vi "HTTP parse headers.vi"(11 "HTTP headers":string="HTTP/1.1 409 Conflict\r\nAccess-Control-Allow-Headers: Origin, X-Requested-With, Content-Type, Accept\r\nAccess-Control-Allow-Methods: GET, POST, PUT, DELETE\r\nAccess-Control-Allow-Origin: *\r\nAccess-Control-Max-Age: 2592000\r\nContent-Type: text/plain\r\nX-Influxdb-Version: InfluxDB v0.8.8 (git: afde71e) (leveldb: 1.15)\r\nDate: Thu, 23 Apr 2015 18:50:38 GMT\r\nContent-Length: 21\r\n\r\n") -> (1 "Status":string, 2 "Status code":string, 3 "HTTP version":string)   [LabVIEW 2013, in "InfluxDB Client.lvclass"]
doc: "Parse HTTP headers to retrieve status information."
uses:
  InfluxDB Client.lvclass
  <vilib>/regexp/Match Regular Expression.xnode
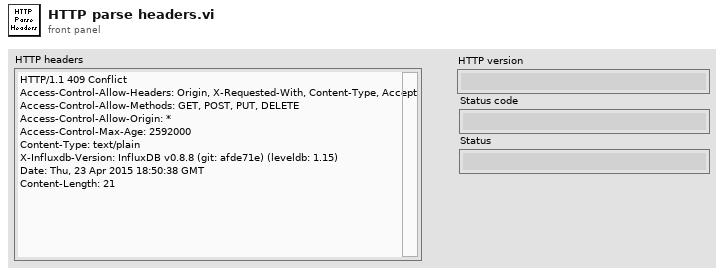
[diagram p1: front panel]
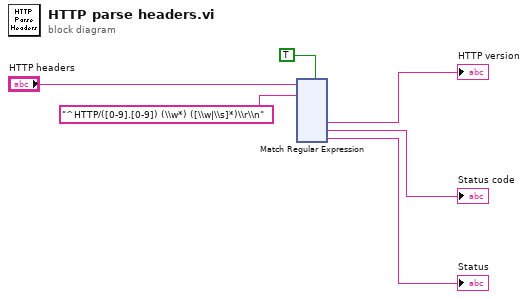
[diagram p0: block diagram]
diagram:
  n1 = xnode "Match Regular Expression"("input string"="HTTP headers", "regular expression"="^HTTP/([0-9].[0-9]) (\\w*) ([\\w|\\s]*)\\r\\n", "multiline? (F)"=TRUE) -> ("submatch 1"=→"HTTP version":string, "submatch 2"=→"Status code":string, "submatch 3"=→"Status":string)  [unwired: 3 in, 5 out]
